vi "__MergeNameMap.vi"(6 "If exist? Skip(T)/Overwrite(F)":bool=TRUE, 8 "error in (no error)":errorcluster, 10 "NameMap B":T1, 11 "NameMap A":T1) -> (0 "error out":errorcluster, 3 "NameMap A after B->A":T1)   [LabVIEW 2019, in "lv-apt-json-file.lvlib"]
uses:
  lv-apt-json-file.lvlib
  Typedef/Def-AttrMap -- NameMap.ctl
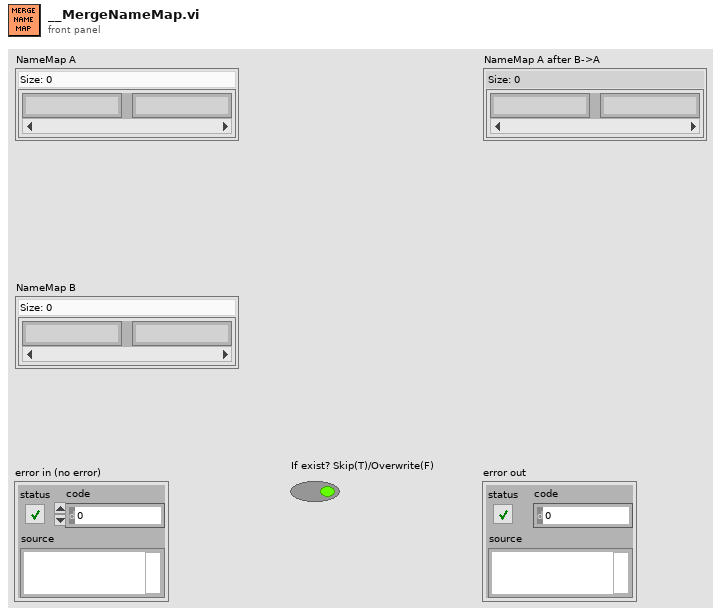
[diagram p1: front panel]
types:
  T1 = typedef "lv-apt-json-file.lvlib/Def-AttrMap -- NameMap.ctl" = map{string, string}
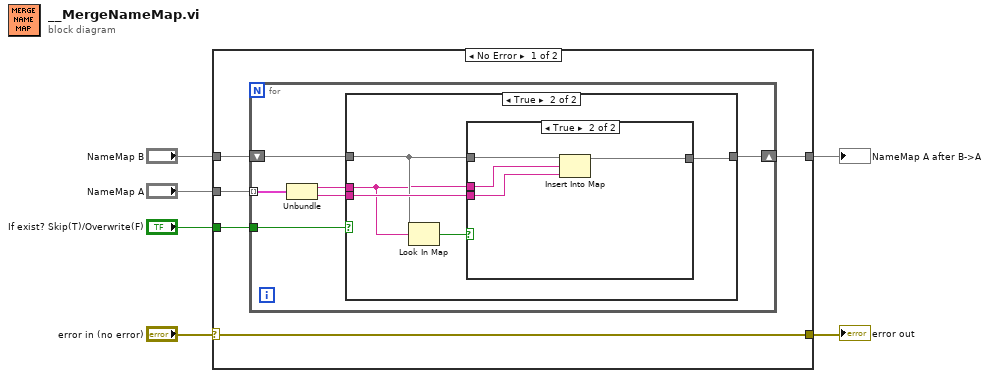
[diagram p0: block diagram]
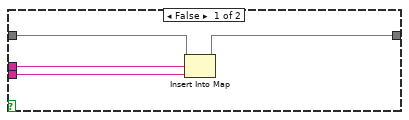
[diagram p2: hidden frame]
diagram:
  n1 = case shown="No Error" "error in (no error)" {
    selector: "error in (no error)" -> [w7 w33]
    tunnel: "NameMap A" -> [w10 w32]
    tunnel: "NameMap B" -> [w11 _]
    tunnel: "If exist? Skip(T)/Overwrite(F)" -> [w9 _]
    tunnel: [w7 w33] -> w2
    tunnel: [w8 w32] -> w1
    frame No Error {
      n2 = for {
        tunnel: w10 -> [w15] mode=indexing
        shift-right: [w12] -> w8
        shift-left: w11 -> [w16]
        tunnel: w9 -> [w17]
        n3 = Unbundle(w15) -> (w14:string, w13:string)
        n4 = case shown="True" w17 {
          tunnel: w16 -> [w21 w24]
          tunnel: w14 -> [w20 w22]
          tunnel: w13 -> [w19 w25]
          tunnel: [w18 w23] -> w12
          frame False {
            n5 = Insert Into Map(map in=w21, key=w20, value=w19) -> (map out=w18:T1)  [unwired: 2 out]
          }
          frame True {
            n6 = Look In Map(map=w24, key=w22) -> (key not found?=w26:bool)  [unwired: 1 in, 1 out]
            n7 = case shown="True" w26 {
              tunnel: w25 -> [_ w29]
              tunnel: w24 -> [w27 w31]
              tunnel: [w27 w30] -> w23
              tunnel: w22 -> [_ w28]
              frame False {
              }
              frame True {
                n8 = Insert Into Map(map in=w31, key=w28, value=w29) -> (map out=w30:T1)  [unwired: 2 out]
              }
            }
          }
        }
      }
    }
    frame Error {
    }
  }
  "NameMap A after B->A" <- w1
  "error out" <- w2
